vi "DAQmx Read (Power 1D DBL NChan 1Samp).vi"(0 "task/channels in":refnum<k21>, 9 "timeout":dbl=10.0 format="%0.2f", 11 "error in":errorcluster) -> (4 "task out":refnum<k21>, 6 "voltage":dbl[](array[numeric]), 8 "current":dbl[](array[numeric]), 15 "error out":errorcluster)   [LabVIEW 2022 SP3]
doc: "Reads one floating-point sample from a task that contains one or more power channels."
uses:
  nilvaiu.dll
panel:
  # "channel"
  # "channel"
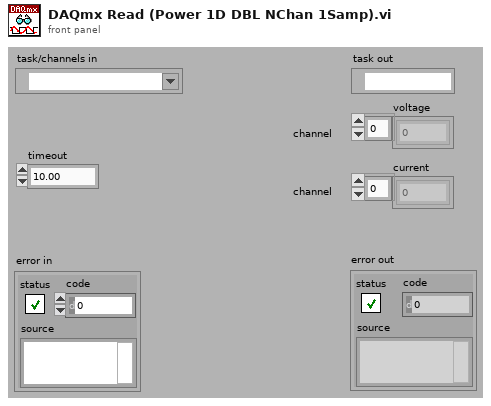
[diagram p1: front panel]
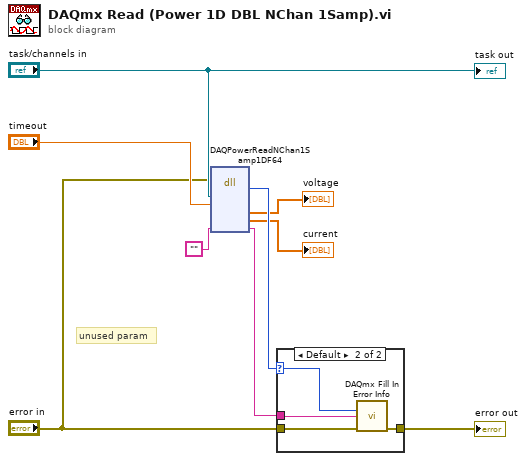
[diagram p0: block diagram]
diagram:
  # "unused param"
  n1 = dll-call lib="nilvaiu.*" fn="DAQPowerReadNChan1Samp1DF64"(error in="error in", "taskID"="task/channels in", "timeout"="timeout", "extendedErrorInfo"="") -> ("return type"=w7:i32, "voltage"=→"voltage":dbl[], "current"=→"current":dbl[], "extendedErrorInfo"=w5:string)  [unwired: 4 in, 4 out]
  n2 = case shown="Default" w7 {
    selector: w7 -> [_ w12]
    tunnel: "error in" -> [w10 w14]
    tunnel: [w10 w13] -> w9
    tunnel: w5 -> [_ w11]
    frame 0 {
    }
    frame Default {
      n3 = call "DAQmx Fill In Error Info.vi"("status code"=w12, "extended error info"=w11, "error in"=w14) -> ("error out"=w13:errorcluster)  [unwired: 1 in, 11 out]
    }
  }
  "error out" <- w9
  "task out" <- "task/channels in"
